vi "Write Toggle Key Binding.vi"(8 "error in (no error)":errorcluster, 10 "ToggleKeyBind":T1, 11 "Boolean.lvclass in":refnum<class "Boolean.lvclass">) -> (0 "error out":errorcluster, 3 "Boolean.lvclass out":refnum<class "Boolean.lvclass">)   [LabVIEW 2015, in "Boolean.lvclass"]
uses:
  Boolean.lvclass
  <vilib>/Utility/miscctls.llb/LVKeyTypeDef.ctl
  Boolean.lvclass/Boolean.ctl
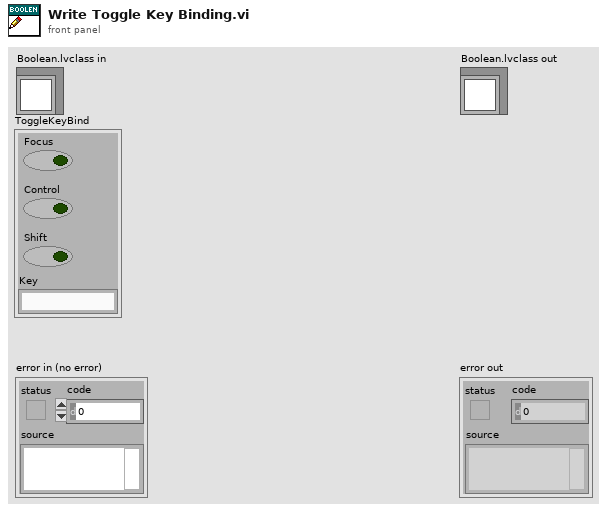
[diagram p1: front panel]
types:
  T1 = typedef "LVKeyTypeDef.ctl" = cluster{"Focus":bool, "Control":bool, "Shift":bool, "Key":string}
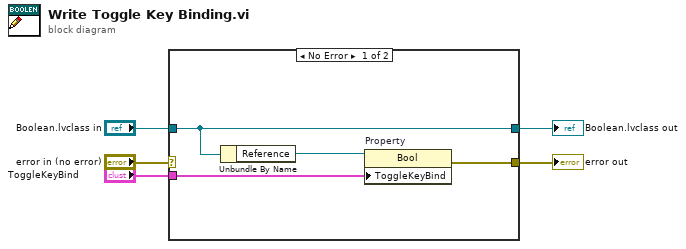
[diagram p0: block diagram]
diagram:
  n1 = case shown="No Error" "error in (no error)" {
    selector: "error in (no error)" -> [_ w11]
    tunnel: [w9 w11] -> w4
    tunnel: [w7 w10] -> w2
    tunnel: "Boolean.lvclass in" -> [w7 w10]
    tunnel: "ToggleKeyBind" -> [w8 _]
    frame No Error {
      n2 = Unbundle By Name(w7) -> ("Reference"=w6:refnum<vi>)
      n3 = property on="Property" class="Bool"(reference=w6, "ToggleKeyBind"=w8) -> (error out=w9:errorcluster)  [unwired: 1 in, 1 out]
    }
    frame Error {
    }
  }
  "error out" <- w4
  "Boolean.lvclass out" <- w2
